vi "Read Overlays.vi"(8 "error in (no error)":errorcluster, 11 "Layered Shape in":refnum<class "Layered Shape.lvclass">) -> (0 "error out":errorcluster, 2 "Overlays":refnum<class "Shape.lvclass">[](array[class]), 3 "Layered Shape out":refnum<class "Layered Shape.lvclass">)   [LabVIEW 2017, in "LV Image Editor Framework.lvlib" / "Layered Shape.lvclass"]
uses:
  Layered Shape.lvclass
  Shape/Shape.lvclass
  Layered Shape.lvclass/Layered Shape.ctl
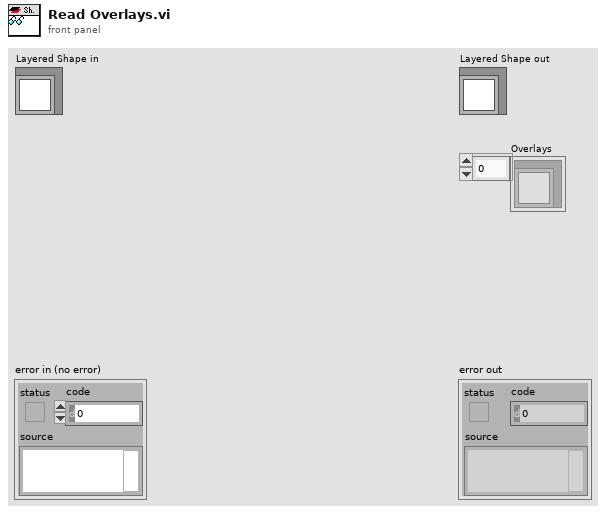
[diagram p1: front panel]
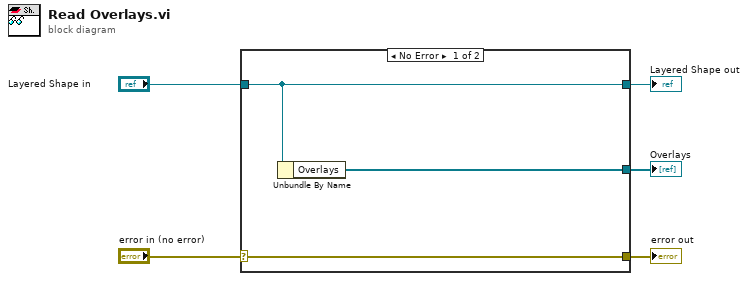
[diagram p0: block diagram]
diagram:
  n1 = case shown="No Error" "error in (no error)" {
    selector: "error in (no error)" -> [w8 w9]
    tunnel: [w8 w9] -> w4
    tunnel: [w7 w10] -> w2
    tunnel: "Layered Shape in" -> [w7 w10]
    tunnel: [w6 _] -> w1
    frame No Error {
      n2 = Unbundle By Name(w7) -> ("Overlays"=w6:refnum<class "Shape.lvclass">[])
    }
    frame Error {
    }
  }
  "error out" <- w4
  "Layered Shape out" <- w2
  "Overlays" <- w1
